vi "Carrier.vi"(6 "Sampling Info (10kS/s)":cluster{"Fs":dbl, "#s":dbl}={"Fs"=10000.0, "#s"=10000.0} {"Fs" format="%.2p"}, 8 "error in (no error)":errorcluster, 10 "Carrier Amplitude (1V)":dbl=1.0, 11 "Carrier Frequency (1kHz)":dbl=1000.0) -> (0 "error out":errorcluster, 2 "Shifted Carrier":waveform(dbl), 3 "Carrier":waveform(dbl))   [LabVIEW 2020]
uses:
  <vilib>/measure/NI_MABase.lvlib
  <vilib>/Analysis/NI_AALPro.lvlib
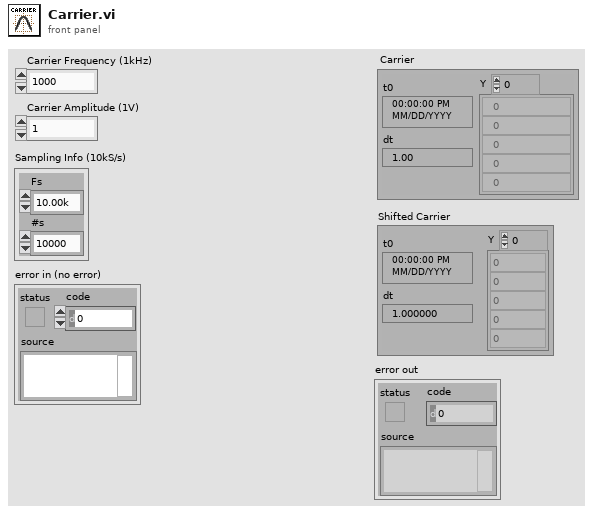
[diagram p1: front panel]
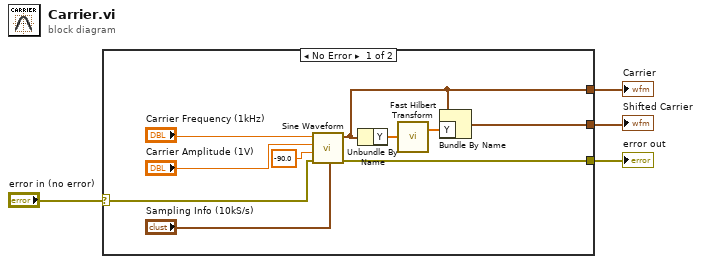
[diagram p0: block diagram]
diagram:
  n1 = case shown="No Error" "error in (no error)" {
    selector: "error in (no error)" -> [w8 w15]
    tunnel: [w7 w15] -> w3
    tunnel: [w6 _] -> w2
    tunnel: [w5 _] -> w1
    frame No Error {
      n2 = call <vilib>:"Sine Waveform.vi"("sampling info"="Sampling Info (10kS/s)", "error in (no error)"=w8, "phase"=-90.0 ("amplitude"), "amplitude"="Carrier Amplitude (1V)", "frequency"="Carrier Frequency (1kHz)") -> ("error out"=w7:errorcluster, "signal out"=w6:waveform(dbl))  [unwired: 5 in]
      n3 = Unbundle By Name(w6) -> ("Y"=w13:dbl[])
      n4 = call <vilib>:"Fast Hilbert Transform.vi"("X"=w13) -> ("Hilbert{X}"=w12:dbl[])  [unwired: 1 out]
      n5 = Bundle By Name(cluster=w6, "Y"=w12) -> (w5:waveform(dbl))
    }
    frame Error {
    }
  }
  "error out" <- w3
  "Shifted Carrier" <- w1
  "Carrier" <- w2
